vi "Draw_box.vi"(6 "Z Value":dbl, 7 "3D?":bool=TRUE, 8 "Top":cluster{"x":dbl, "y":dbl}[][](array[cluster]), 9 "element":cluster{"row":i32, "col":i32}, 10 "Base":cluster{"x":dbl, "y":dbl}[][](array[cluster]), 11 "picture in":picture) -> (1 "base":cluster{"x":dbl, "y":dbl}[](array[cluster]), 3 "picture out":picture)   [LabVIEW 2022 SP3]
panel:
  out "top":cluster{"x":dbl, "y":dbl}[](array[cluster])
  out "right face":cluster{"x":dbl, "y":dbl}[](array[cluster])
  out "left face":cluster{"x":dbl, "y":dbl}[](array[cluster])
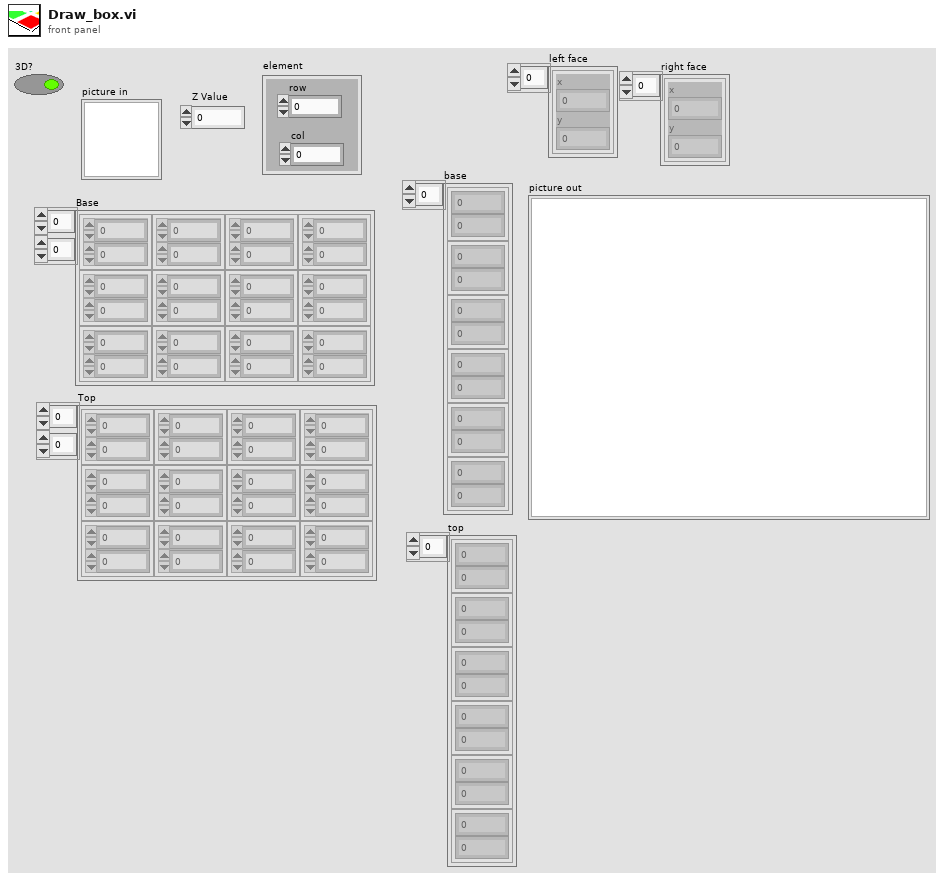
[diagram p1: front panel]
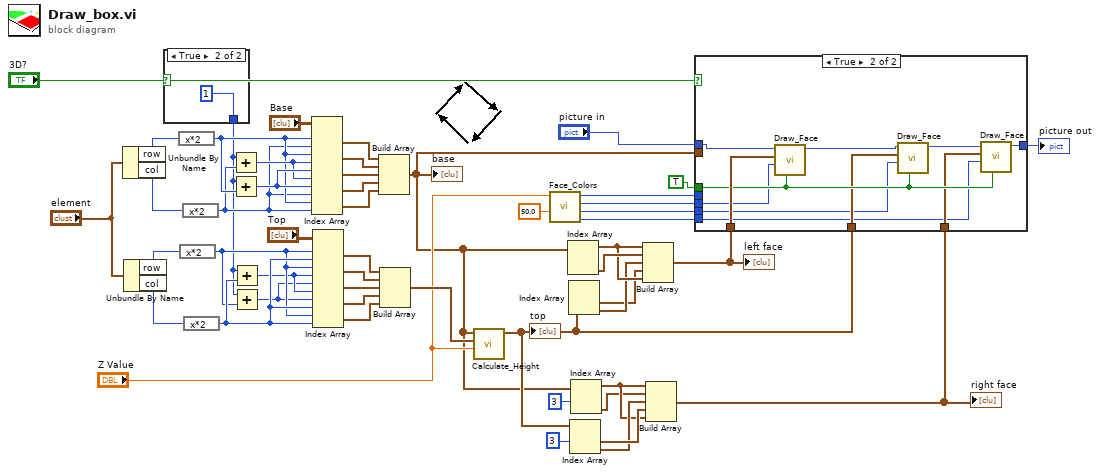
[diagram p0: block diagram]
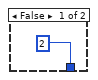
[diagram p2: hidden frame]
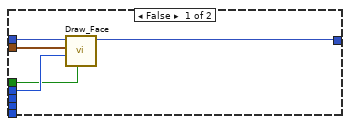
[diagram p3: hidden frame]
diagram:
  n1 = Unbundle By Name("element") -> ("row"=w43:i32, "col"=w42:i32)
  n2 = Unbundle By Name("element") -> ("row"=w37:i32, "col"=w38:i32)
  n3 = case shown="True" "3D?" {
    tunnel: [2 1] -> w2
    frame False {
    }
    frame True {
    }
  }
  n4 = expression code="x*2"(w43) -> (w45:i32)
  n5 = expression code="x*2"(w37) -> (w35:i32)
  n6 = expression code="x*2"(w42) -> (w44:i32)
  n7 = expression code="x*2"(w38) -> (w36:i32)
  n8 = Add(x=w2, y=w44) -> (x+y=w46:i32)
  n9 = Add(x=w2, y=w45) -> (x+y=w47:i32)
  n10 = Add(x=w2, y=w36) -> (x+y=w34:i32)
  n11 = Add(x=w2, y=w35) -> (x+y=w33:i32)
  n12 = Index Array(array="Base", index (row) #1=w45, index (col) #1=w44, index (row) #2=w45, index (col) #2=w46, index (row) #3=w47, index (col) #3=w46, index (row) #4=w47, index (col) #4=w44, index (row) #5=w45, index (col) #5=w44) -> (element #1=w51:cluster{"x":dbl, "y":dbl}, element #2=w48:cluster{"x":dbl, "y":dbl}, element #3=w49:cluster{"x":dbl, "y":dbl}, element #4=w50:cluster{"x":dbl, "y":dbl}, element #5=w40:cluster{"x":dbl, "y":dbl})
  n13 = Index Array(array="Top", index (row) #1=w35, index (col) #1=w36, index (row) #2=w35, index (col) #2=w34, index (row) #3=w33, index (col) #3=w34, index (row) #4=w33, index (col) #4=w36, index (row) #5=w35, index (col) #5=w36) -> (element #1=w29:cluster{"x":dbl, "y":dbl}, element #2=w32:cluster{"x":dbl, "y":dbl}, element #3=w31:cluster{"x":dbl, "y":dbl}, element #4=w30:cluster{"x":dbl, "y":dbl}, element #5=w39:cluster{"x":dbl, "y":dbl})
  n14 = Build Array(w51, w48, w49, w50, w40) -> (w4:cluster{"x":dbl, "y":dbl}[])
  "base" <- w4
  n15 = Build Array(w29, w32, w31, w30, w39) -> (w13:cluster{"x":dbl, "y":dbl}[])
  n16 = call "Calculate_Height.vi"("Z Value"="Z Value", "Full top"=w13, "Base"=w4) -> ("Adjusted top"=w12:cluster{"x":dbl, "y":dbl}[])  [unwired: 8 in]
  "top" <- w12
  n17 = call "Face_Colors.vi"("offset"=50.0, "Z Value"="Z Value") -> ("right"=w8:u32, "top"=w9:u32, "left"=w10:u32, "bottom"=w5:u32)  [unwired: 6 in]
  n18 = Index Array(array=w4) -> (element #1=w25:cluster{"x":dbl, "y":dbl}, element #2=w26:cluster{"x":dbl, "y":dbl})  [unwired: 2 in]
  n19 = Index Array(array=w12) -> (element #1=w22:cluster{"x":dbl, "y":dbl}, element #2=w23:cluster{"x":dbl, "y":dbl})  [unwired: 2 in]
  n20 = Index Array(array=w12, index #1=3 ("index")) -> (element #1=w21:cluster{"x":dbl, "y":dbl}, element #2=w20:cluster{"x":dbl, "y":dbl})  [unwired: 1 in]
  n21 = Index Array(array=w4, index #1=3 ("index")) -> (element #1=w19:cluster{"x":dbl, "y":dbl}, element #2=w18:cluster{"x":dbl, "y":dbl})  [unwired: 1 in]
  n22 = Build Array(w25, w26, w23, w22, w25) -> (w24:cluster{"x":dbl, "y":dbl}[])
  "left face" <- w24
  n23 = Build Array(w19, w18, w20, w21, w19) -> (w14:cluster{"x":dbl, "y":dbl}[])
  "right face" <- w14
  n24 = case shown="True" "3D?" {
    tunnel: w24 -> [_ w68]
    tunnel: [w55 w67] -> w15
    tunnel: TRUE ("fill?(F)") -> [w54 w65]
    tunnel: w14 -> [_ w64]
    tunnel: w12 -> [_ w63]
    tunnel: w10 -> [_ w62]
    tunnel: w9 -> [_ w61]
    tunnel: w8 -> [_ w60]
    tunnel: w5 -> [w58 _]
    tunnel: w4 -> [w57 _]
    tunnel: "picture in" -> [w56 w59]
    frame False {
      n25 = call "Draw_Face.vi"("fill?(F)"=w54, "color"=w58, "Array"=w57, "picture in"=w56) -> ("new picture"=w55:picture)  [unwired: 7 in]
    }
    frame True {
      n26 = call "Draw_Face.vi"("fill?(F)"=w65, "color"=w62, "Array"=w68, "picture in"=w59) -> ("new picture"=w69:picture)  [unwired: 7 in]
      n27 = call "Draw_Face.vi"("fill?(F)"=w65, "color"=w61, "Array"=w63, "picture in"=w69) -> ("new picture"=w66:picture)  [unwired: 7 in]
      n28 = call "Draw_Face.vi"("fill?(F)"=w65, "color"=w60, "Array"=w64, "picture in"=w66) -> ("new picture"=w67:picture)  [unwired: 7 in]
    }
  }
  "picture out" <- w15
